vi "Read Variables.vi"(8 "error in (no error)":errorcluster, 9 "Slide Refnum":refnum<vi>, 10 "Ctl Refnum":refnum<vi>, 11 "Worksheet Reference":refnum<k7>) -> (0 "error out":errorcluster)   [LabVIEW 2015]
uses:
  Variable cluster.ctl
panel:
  in  "Variable Clusters":T1
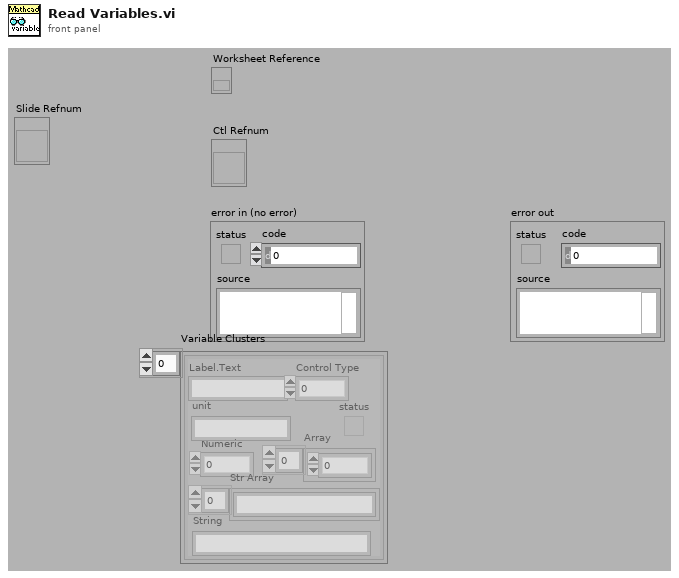
[diagram p1: front panel]
types:
  T1 = typedef "Variable cluster.ctl" = cluster{"Label.Text":string, "Control Type":u32, "Numeric":dbl, "Array":dbl[], "status":bool, "Str Array":string[], "String":string, "unit":string}[]
  T2 = cluster{"Label.Text":string, "Control Type":u32, "Numeric":dbl, "Array":dbl[], "status":bool, "Str Array":string[], "String":string, "unit":string}
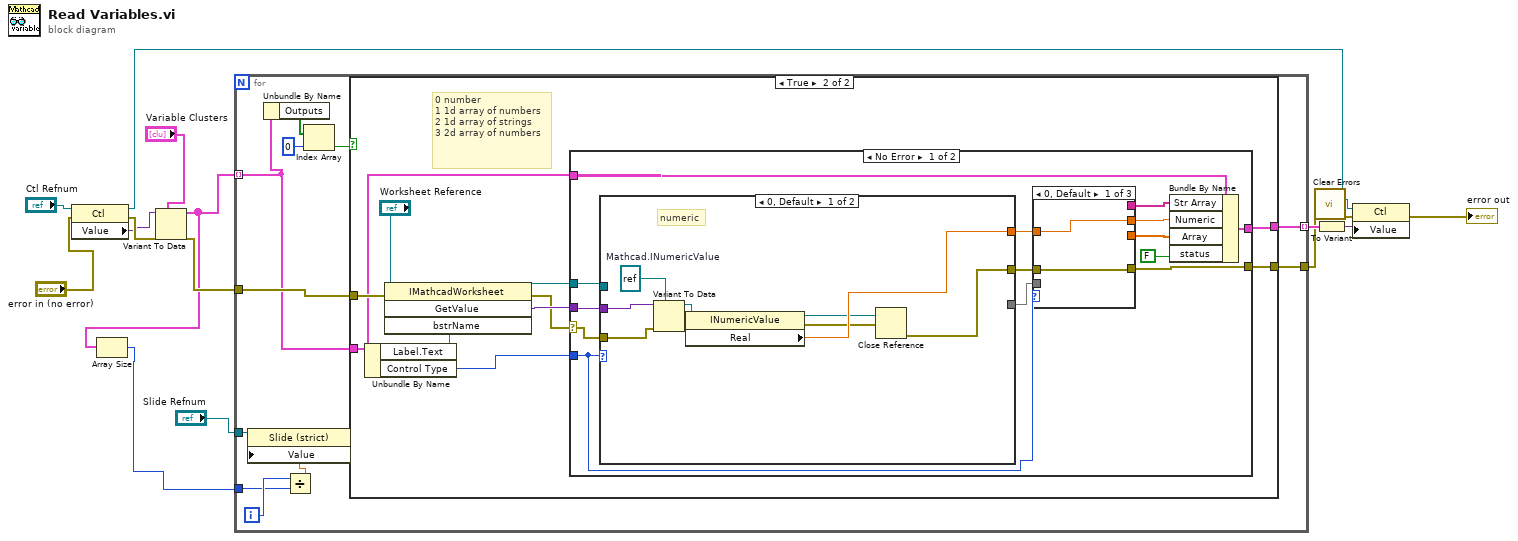
[diagram p0: block diagram]
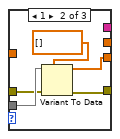
[diagram p3: hidden frame]
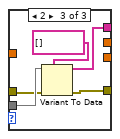
[diagram p4: hidden frame]
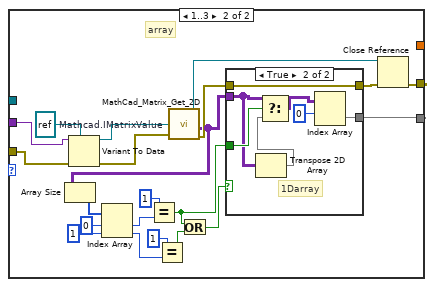
[diagram p5: hidden frame]
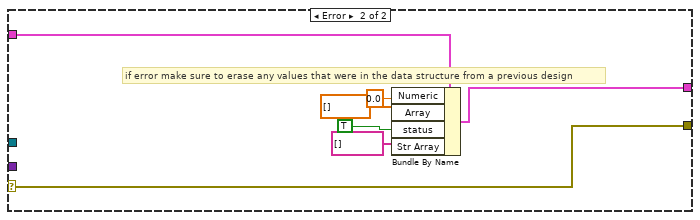
[diagram p7: hidden frame]
diagram:
  n1 = property class="Ctl"(reference="Ctl Refnum", error in="error in (no error)") -> (reference out=w7:refnum<vi>, error out=w14:errorcluster, "Value"=w13:variant)
  n2 = Variant To Data(error in=w14, type="Variable Clusters", Variant=w13) -> (data=w3:T1, error out=w10:errorcluster)
  n3 = Array Size(array=w3) -> (size(s)=w1:i32)
  n4 = for {
    tunnel: w10 -> [w26]
    tunnel: [w25] -> w6
    tunnel: w3 -> [w23] mode=indexing
    tunnel: [w24] -> w9 mode=indexing
    tunnel: "Slide Refnum" -> [w19]
    tunnel: w1 -> [w16]
    i -> [w17]
    n5 = Unbundle By Name(w23) -> ("Outputs"=w22:bool[])
    n6 = Divide(x=w17, y=w16) -> (x/y=w18:dbl)
    n7 = property class="Slide (strict)"(reference=w19, "Value"=w18) -> ()  [unwired: 1 in, 2 out]
    n8 = Index Array(array=w22, index=0) -> (element=w20:bool)
    n9 = case shown="True" w20 {
      tunnel: w26 -> [w28 w38]
      tunnel: [w28 w37] -> w25
      tunnel: [w27 w36] -> w24
      tunnel: w23 -> [w27 w29]
      frame False {
        # "Don't return this value to user"
      }
      frame True {
        # "0\tnumber\n1\t1d array of numbers\n2\t1d array of strings\n3\t2d array of numbers"
        n10 = Unbundle By Name(w29) -> ("Label.Text"=w32:string, "Control Type"=w31:u32)
        n11 = invoke class="IMathcadWorksheet" method="GetValue"(reference="Worksheet Reference", error in=w38, "bstrName"=w32) -> (reference out=w33:refnum<k7>, error out=w30:errorcluster, "GetValue"=w34:variant)  [unwired: 1 in, 1 out]
        n12 = case shown="No Error" w30 {
          selector: w30 -> [w48 w106]
          tunnel: w34 -> [w52 _]
          tunnel: w33 -> [w51 _]
          tunnel: w31 -> [w46 _]
          tunnel: w29 -> [w50 w109]
          tunnel: [w40 w106] -> w37
          tunnel: [w49 w108] -> w36
          frame No Error {
            n13 = case shown="0, Default" w46 {
              tunnel: w52 -> [w73 w93]
              tunnel: w48 -> [w72 w94]
              tunnel: w51 -> [_ _]
              tunnel: [w69 w90] -> w39
              tunnel: [w68 _] -> w42
              tunnel: [_ w75] -> w45
              frame 0, Default {
                w71 = refnum<k7> refnum  # Mathcad.INumericValue
                # "numeric"
                n14 = Variant To Data(error in=w72, type=w71, Variant=w73) -> (data=w70:refnum<k7>, error out=w66:errorcluster)
                n15 = property class="INumericValue"(reference=w70, error in=w66) -> (reference out=w65:refnum<k7>, error out=w67:errorcluster, "Real"=w68:dbl)
                n16 = Close Reference(reference=w65, error in (no error)=w67) -> (error out=w69:errorcluster)
              }
              frame 1..3 {
                w92 = refnum<k7> refnum  # Mathcad.IMatrixValue
                # "array"
                n17 = Variant To Data(error in=w94, type=w92, Variant=w93) -> (data=w91:refnum<k7>, error out=w87:errorcluster)
                n18 = call "MathCad_Matrix_Get_2D.vi"("Mathcad.IMatrixValue Refnum"=w91, "error out 2"=w87) -> ("Mathcad.IMatrixValue Refnum"=w89:refnum<k7>, "Array"=w86:variant[][], "error out"=w88:errorcluster)  [unwired: 2 in]
                n19 = Array Size(array=w86) -> (size(s)=w85:i32[])
                n20 = Index Array(array=w85, index #1=0 ("index"), index #2=1 ("index")) -> (element #1=w82:i32, element #2=w79:i32)
                n21 = Equal?(x=1 ("index"), y=w82) -> (x = y?=w76:bool)
                n22 = Equal?(x=1 ("index"), y=w79) -> (x = y?=w78:bool)
                n23 = Or(x=w76, y=w78) -> (x .or. y?=w77:bool)
                n24 = case shown="True" w77 {
                  tunnel: w88 -> [w95 w96]
                  tunnel: w86 -> [_ w99]
                  tunnel: w76 -> [_ w101]
                  tunnel: [_ w97] -> w75
                  tunnel: [w95 w96] -> w74
                  frame False {
                    # "2Darray"
                  }
                  frame True {
                    # "1Darray"
                    n25 = Transpose 2D Array(2D array=w99) -> (transposed array=w98:variant[][])
                    n26 = Select(t=w99, s=w101, f=w98) -> (s? t:f=w100:variant[][])
                    n27 = Index Array(array=w100, index (row)=0) -> (element=w97:variant[])  [unwired: 1 in]
                  }
                }
                n28 = Close Reference(reference=w89, error in (no error)=w74) -> (error out=w90:errorcluster)
              }
            }
            n29 = case shown="0, Default" w46 {
              tunnel: w45 -> [_ w59 w64]
              tunnel: [_ w57 _] -> w44
              tunnel: [w54 _ _] -> w43
              tunnel: w42 -> [w54 _ _]
              tunnel: [_ _ w62] -> w41
              tunnel: [w53 w55 w61] -> w40
              tunnel: w39 -> [w53 w56 w60]
              frame 0, Default {
              }
              frame 1 {
                n30 = Variant To Data(error in=w56, type=dbl[] [] ("Array"), Variant=w59) -> (data=w57:dbl[], error out=w55:errorcluster)
              }
              frame 2 {
                n31 = Variant To Data(error in=w60, type=string[] [] ("Array"), Variant=w64) -> (data=w62:string[], error out=w61:errorcluster)
              }
            }
            n32 = Bundle By Name(cluster=w50, "Str Array"=w41, "Numeric"=w43, "Array"=w44, "status"=FALSE) -> (w49:T2)
          }
          frame Error {
            # "if error make sure to erase any values that were in the data structure from a previous design"
            n33 = Bundle By Name(cluster=w109, "Numeric"=0.0, "Array"=dbl[] [], "status"=TRUE, "Str Array"=string[] []) -> (w108:T2)
          }
        }
      }
    }
  }
  n34 = call <vilib>:"Clear Errors.vi"("error in (no error)"=w6) -> ("error out"=w4:errorcluster)  [unwired: 5 in, 1 out]
  n35 = To Variant(anything=w9) -> (Variant=w8:variant)
  n36 = property class="Ctl"(reference=w7, error in=w4, "Value"=w8) -> (error out=→"error out":errorcluster)  [unwired: 1 out]
